vi "Teleop.vi"(10 "Match Info":T1={"Autonomous Elapsed Seconds"=0.0, "TeleOp Elapsed Seconds"=0.0, "Disabled Elapsed Seconds"=0.0, "Visited Autonomous"=FALSE, "Visited TeleOp"=FALSE, "Visited Disabled"=FALSE, "Autonomous Settings"={"Autonomous Style"=enum."Independent", "VI Refnum"=refnum}}, 11 "Call Context":T2) -> ()   [LabVIEW 2016]
doc: "This VI is called for each TeleOp packet received from the DS where the robot is not disabled. It is often used to read from the joysticks and update I/O or to update setpoints for timed control loops. It should complete and return within 20 milliseconds or it may miss DS packets."
uses:
  <vilib>/Rock Robotics/WPI/Ultrasonic/WPI_SonarSRF04DigitalRefNum Registry Get.vi
  <vilib>/Rock Robotics/WPI/Ultrasonic/WPI_SonarSRF04DigitalGetRange.vi
  <vilib>/gmath/NI_Gmath.lvlib
  <vilib>/Rock Robotics/WPI/Relay/WPI_RelayValue.ctl
  <vilib>/Rock Robotics/WPI/DriverStation/WPI_DriverStationMatch Info.ctl
  <vilib>/Rock Robotics/WPI/DriverStation/WPI_DriverStationDerivedRobotMode.ctl
panel:
  in  "Control Effort":dbl[](array[numeric])=[0.0, 0.0, 0.0, 0.0]
  in  "RPM Array":dbl[](array[numeric])=[0.0, 0.0, 0.0, 0.0]
  out "Encoder Index Count":dbl
  in  "OR Speed":dbl
  in  "Override?":bool
  out "Shooter RPM":dbl
  in  "kP":dbl=1.0 format="%#_13g"
  out "Shooter RPM 2":dbl(graph)
  in  "SET RPM":dbl format="%#_13g"
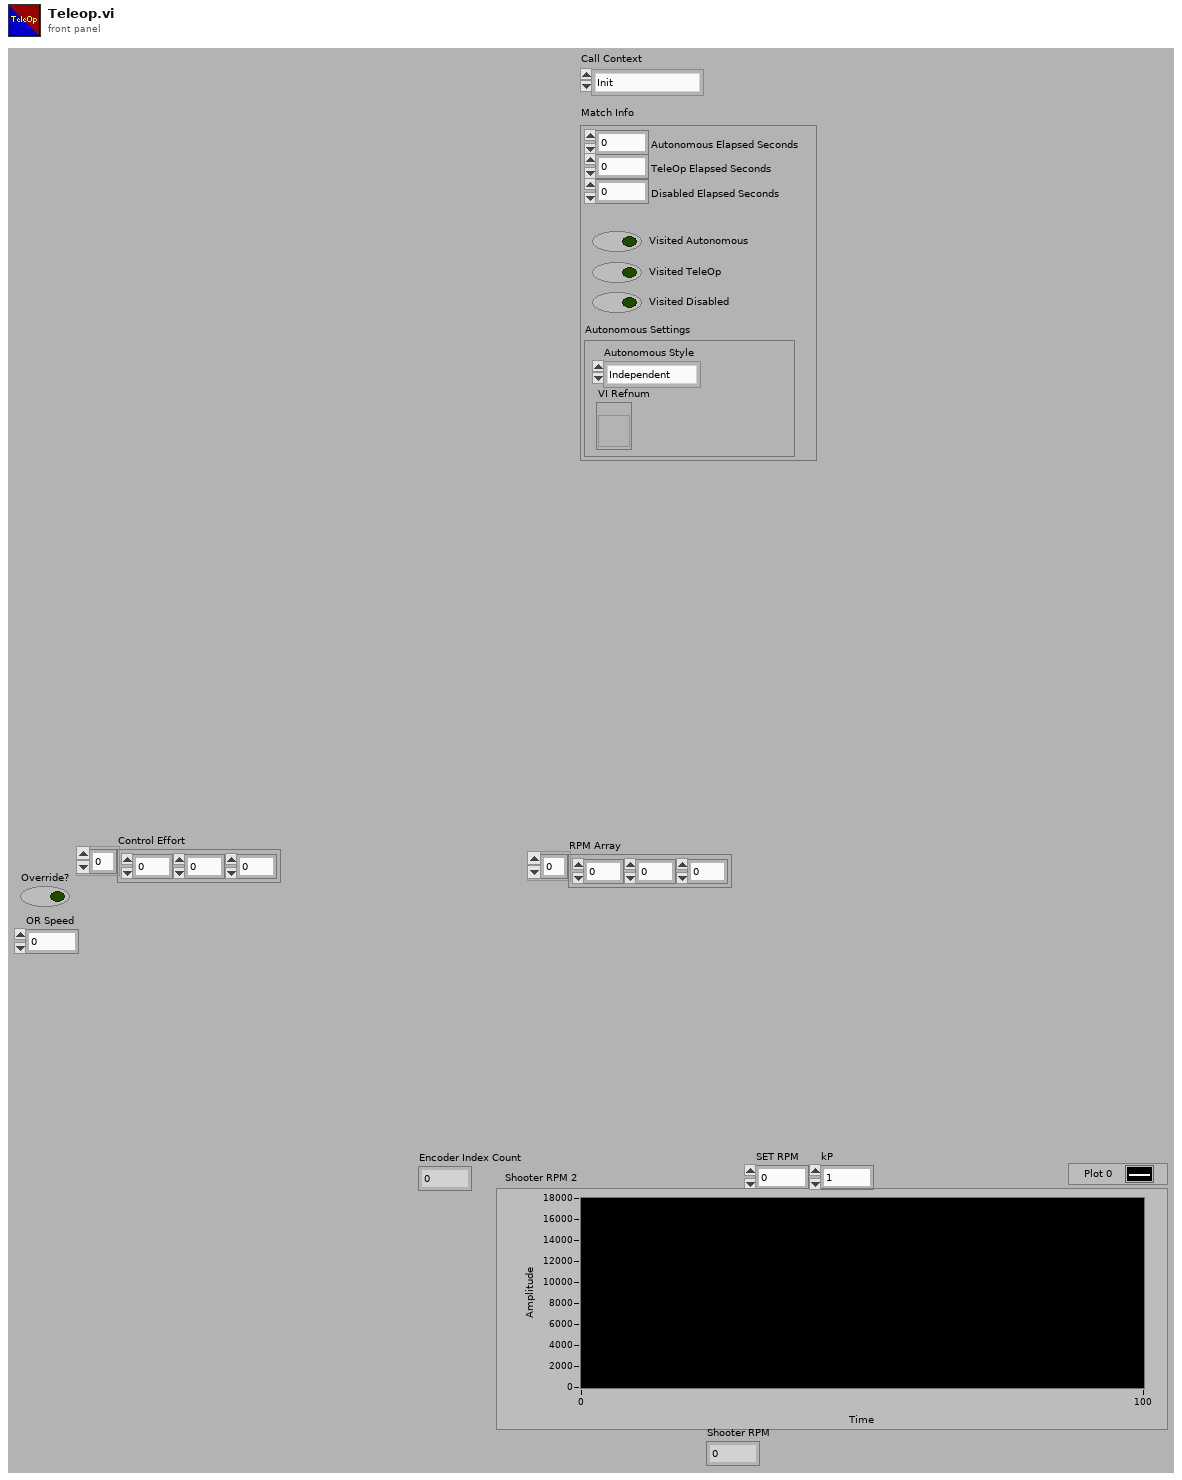
[diagram p1: front panel]
types:
  T1 = typedef "WPI_DriverStationMatch Info.ctl" = cluster{"Autonomous Elapsed Seconds":dbl, "TeleOp Elapsed Seconds":dbl, "Disabled Elapsed Seconds":dbl, "Visited Autonomous":bool, "Visited TeleOp":bool, "Visited Disabled":bool, "Autonomous Settings":cluster{"Autonomous Style":enum16{"Iterative", "Independent"}, "VI Refnum":refnum<vi>}}
  T2 = typedef "WPI_DriverStationDerivedRobotMode.ctl" = enum16{"Init", "Execute", "Stop"}
  T3 = typedef "WPI_JoystickDevRef.ctl" = cluster{"Device":T4}
  T4 = typedef "WPI_JoystickDeviceEnum.ctl" = enum16{"USB 0", "USB 1", "USB 2", "USB 3", "USB 4", "USB 5"}
  T5 = typedef "WPI_MotorControlDeviceRef.ctl" = cluster{"DeviceStatus":errorcluster, "Type":T6, "PWM":cluster{"PWM Channel":T7, "DeadBand":T8}, "CAN":cluster{"Device Number":u8, "SetOutput VI Ref":variant, "GetOutput VI Ref":variant, "Enable VI Ref":variant, "Disable VI Ref":variant, "Data":variant}, "Invert":bool}
  T6 = typedef "WPI_MotorControlType.ctl" = enum16{"PWM", "CAN"}
  T7 = typedef "FPGA_DIOPWMChannel.ctl" = enum8{"PWM 0", "PWM 1", "PWM 2", "PWM 3", "PWM 4", "PWM 5", "PWM 6", "PWM 7", "PWM 8", "PWM 9", "PWM MXP 0", "PWM MXP 1", "PWM MXP 2", "PWM MXP 3", "PWM MXP 4", "PWM MXP 5", "PWM MXP 6", "PWM MXP 7", "PWM MXP 8", "PWM MXP 9", "Invalid"}
  T8 = typedef "WPI_PWMDeadband.ctl" = cluster{"Name":string, "maxPositivePwm":i32, "minPositivePwm":i32, "centerPwm":i32, "maxNegativePwm":i32, "minNegativePwm":i32, "angularRange":u16}
  T9 = typedef "WPI_CANTalonSRX_GlobalStatus.ctl" = cluster{"Applied Throttle":dbl, "Module Enabled":bool, "CAN Error":errorcluster, "Closed Loop Error":dbl, "Forward Limit Switch Closed":bool, "Reverse Limit Switch Closed":bool, "Sensor Position":dbl, "Sensor Velocity":dbl, "Current":dbl, "Sticky Fault - Over Temp":bool, "Sticky Fault - Under Voltage":bool, "Sticky Fault - Forward Limit":bool, "Sticky Fault - Reverse Limit":bool, "Sticky Fault - Forward Soft Limit":bool, "Sticky Fault - Reverse Soft Limit":bool, "Brake is Enabled":bool, "Encoder Position":dbl, "Encoder Velocity":dbl, "Encoder Index Count":dbl, "Encoder A Pin State":bool, "Encoder B Pin State":bool, "Encoder Index Pin State":bool, "Analog In":dbl, "Analog In Velocity":dbl, "Temperature (C)":dbl, "Battery Voltage":dbl, "Control 5 Is Supported":bool, "Current Profile Slot Select":dbl, "Pos Div 8":bool, "Vel Div 4":bool, "Pulse Width Position":i32, "Pulse Width Velocity":i32, "Pulse Width Rise To Rise (us)":i32, "Pulse Width Rise To Fall (us)":i32, "Mot Prof Active Is Under Run":bool, "Mot Prof Active Has Under Run":bool, "Mot Prof Active Is Last":bool, "Mot Prof Active Velocity Only":bool, "Mot Prof Active Is Valid":bool, "Mot Prof Buffer Is Full":bool, "Mot Prof Active Profile Slot Select":i32, "Mot Prof NextID":i32, "Mot Prof Count":i32, "Mot Prof Active Velocity":dbl, "Mot Prof Active Position":dbl, "Mot Prof Output Enable":i32}
  T10 = typedef "WPI_UltrasonicDeviceRef.ctl" = cluster{"DevStatus":errorcluster, "Ping Channel":T11, "Echo Channel":T11, "CntIndex":T12}
  T11 = typedef "FPGA_DIOChannel.ctl" = enum8{"DIO 0", "DIO 1", "DIO 2", "DIO 3", "DIO 4", "DIO 5", "DIO 6", "DIO 7", "DIO 8", "DIO 9", "DIO MXP 0", "DIO MXP 1", "DIO MXP 2", "DIO MXP 3", "DIO MXP 4", "DIO MXP 5", "DIO MXP 6", "DIO MXP 7", "DIO MXP 8", "DIO MXP 9", "DIO MXP 10", "DIO MXP 11", "DIO MXP 12", "DIO MXP 13", "DIO MXP 14", "DIO MXP 15", "SPI Port CS1", "SPI Port CS2", "SPI Port CS3", "SPI Port MISO", "SPI Port MOSI", "Invalid"}
  T12 = typedef "FPGA_CounterCtrSystemIndex.ctl" = enum8{"Ctr 0", "Ctr 1", "Ctr 2", "Ctr 3", "Ctr 4", "Ctr 5", "Ctr 6", "Ctr 7", "Invalid"}
  T13 = typedef "WPI_GyroDevRef.ctl" = cluster{"DevStatus":errorcluster, "Analog Channel":T14, "Offset":dbl, "Gain (VoltsPerDegree/Second)":dbl, "Gyro Type":enum16{"Analog", "XRS450"}, "Handle":i32, "SPI Bus":T15, "Device Found":bool, "Sample Rate":dbl, "Calibrate On Open":bool}
  T14 = typedef "FPGA_AIChannel.ctl" = enum8{"AI 0", "AI 1", "AI 2", "AI 3", "AI MXP 0", "AI MXP 1", "AI MXP 2", "AI MXP 3", "Invalid"}
  T15 = typedef "spi_bus.ctl" = enum16{"SPI On-Board, CS0", "SPI On-Board, CS1", "SPI On-Board, CS2", "SPI On-Board, CS3", "SPI MXP", "Invalid"}
  T16 = typedef "WPI_RelayValue.ctl" = enum16{"Off", "On", "Forward", "Reverse"}
  T17 = typedef "WPI_RelayDevRef.ctl" = cluster{"DevStatus":errorcluster, "Relay Channel":T18, "Relay Direction":T19}
  T18 = typedef "FPGA_DIORelayChannel.ctl" = enum8{"Relay 0", "Relay 1", "Relay 2", "Relay 3", "Invalid"}
  T19 = typedef "WPI_RelayDirection.ctl" = enum16{"Both directions", "Forward only", "Reverse only"}
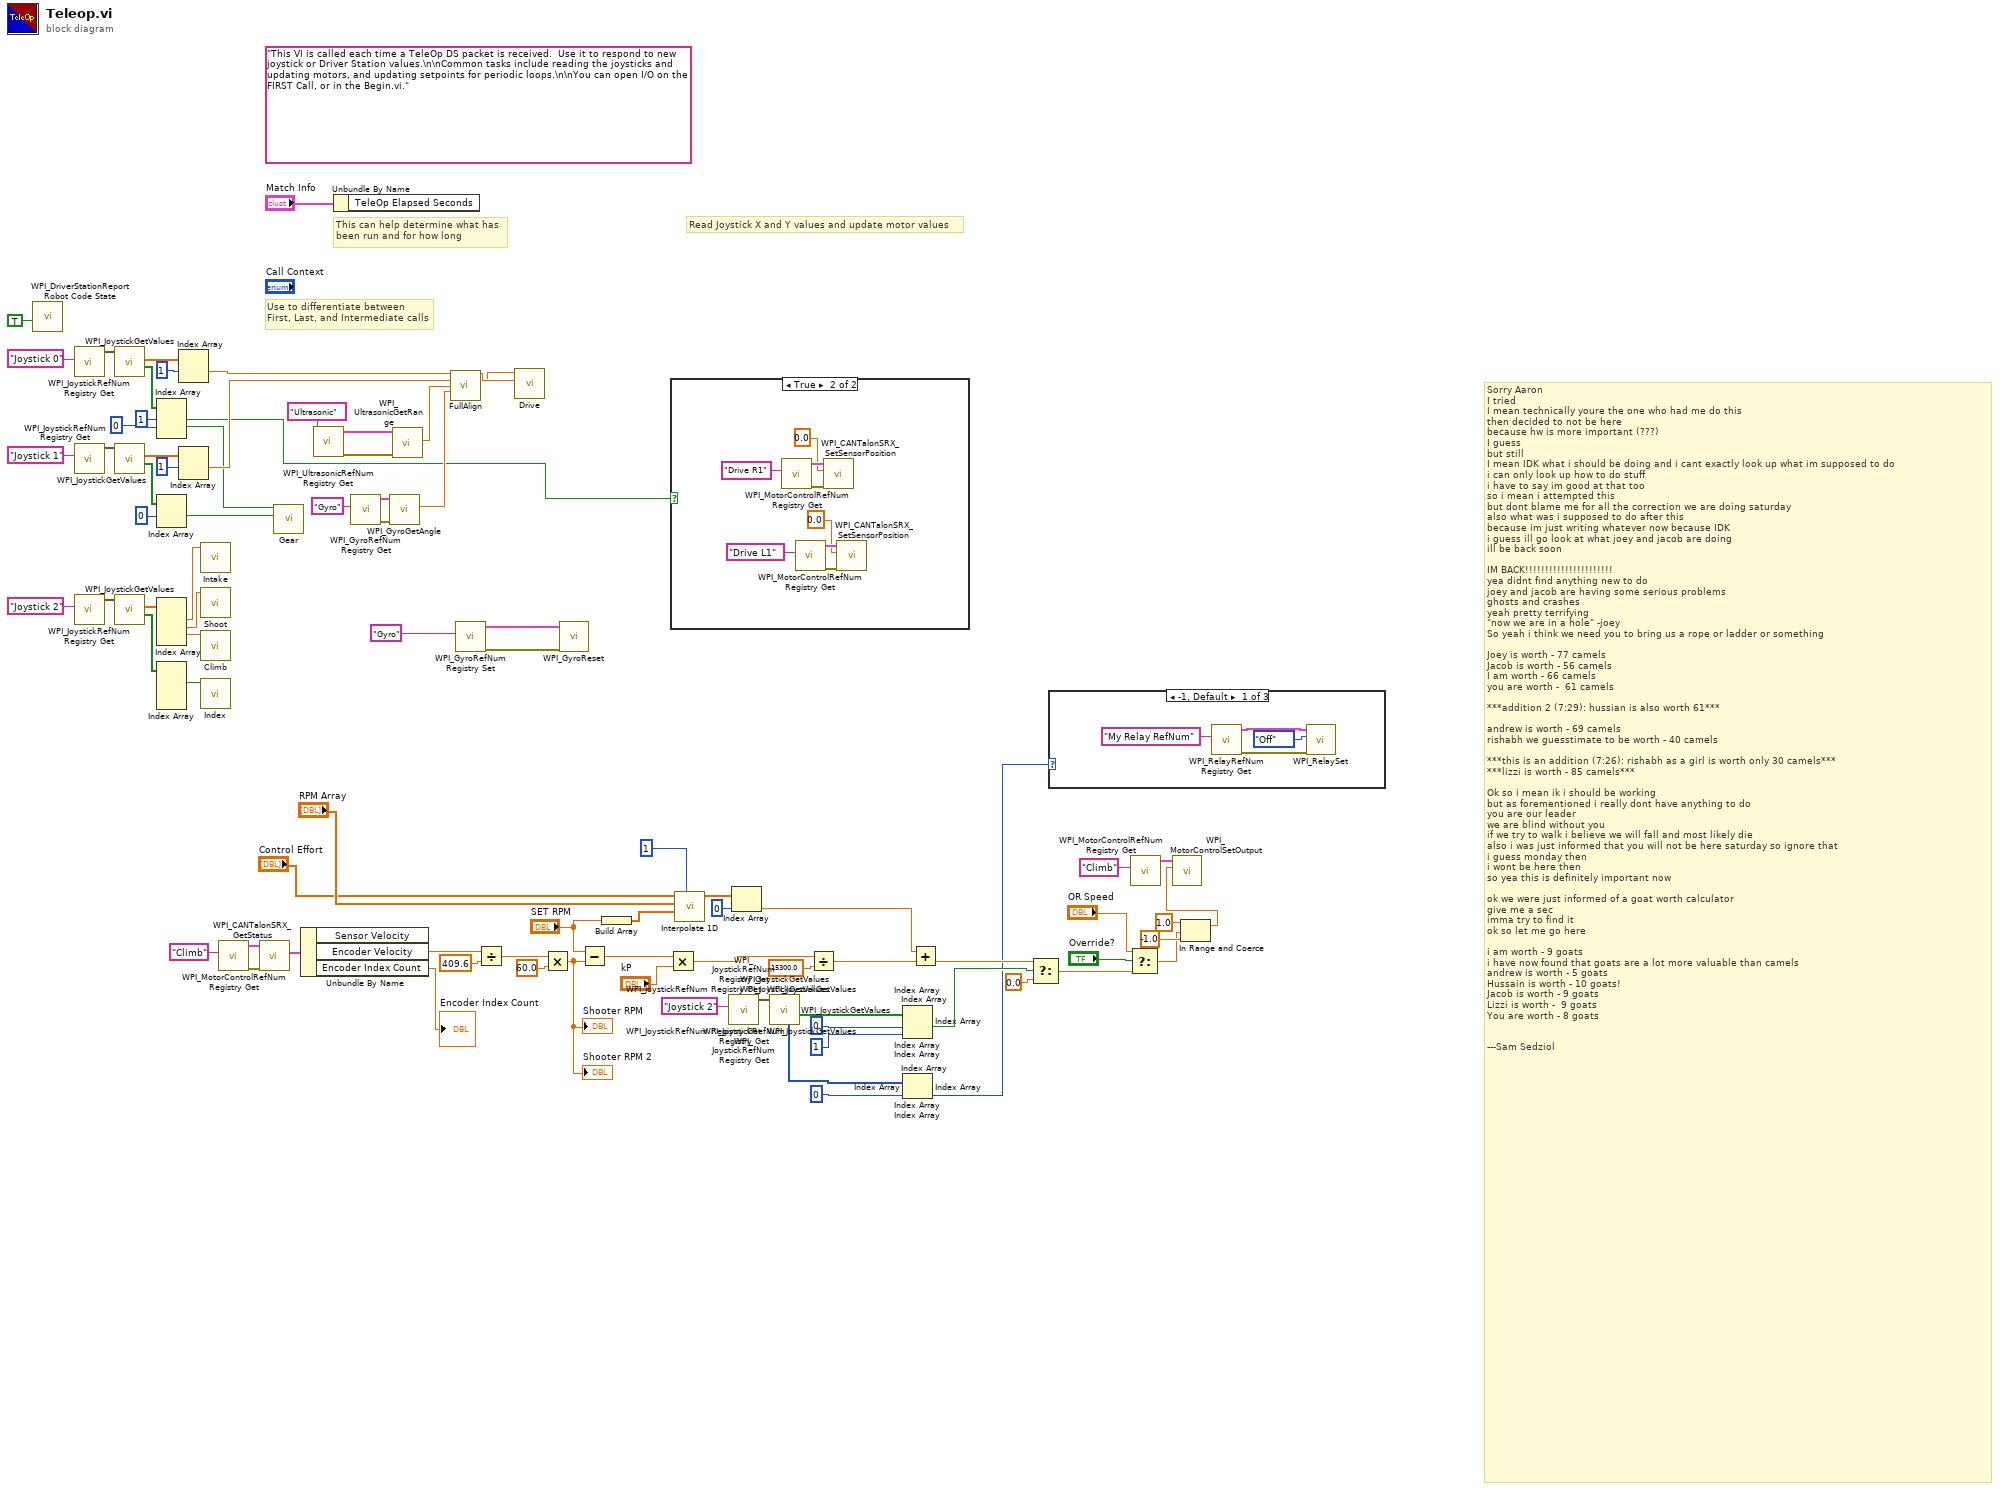
[diagram p0: block diagram]
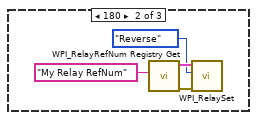
[diagram p3: hidden frame]
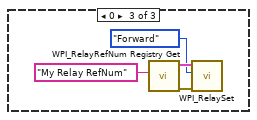
[diagram p4: hidden frame]
diagram:
  (unwired) "This VI is called each time a TeleOp DS packet is received.  Use it to respond to new joystick or Driver Station values.\n\nCommon tasks include reading the joysticks and updating motors, and updating setpoints for periodic loops.\n\nYou can open I/O on the FIRST Call, or in the Begin.vi."
  # "Sorry Aaron\nI tried\nI mean technically youre the one who had me do this\nthen decided to not be here\nbecause hw is more important (???)\nI guess\nbut still\nI mean IDK what i should be doing and i cant exactly look up what im supposed to do\ni can only look up how to do stuff\ni have to say im good at that too\nso i mean i attempted this\nbut dont blame me for all the correction we are doing saturday\nalso what was i supposed to do after this\nbecause im just writing whatever now because IDK\ni guess ill go look at what joey and jacob are doing\nill be back soon\n\nIM BACK!!!!!!!!!!!!!!!!!!!!!!\nyea didnt find anything new to do\njoey and jacob are having some serious problems\nghosts and crashes\nyeah pretty terrifying\n\"now we are in a hole\" -joey\nSo yeah i think we need you to bring us a rope or ladder or something\n\nJoey is worth - 77 camels\nJacob is worth - 56 camels\nI am worth - 66 camels\nyou are worth -  61 camels \n\n***addition 2 (7:29): hussian is also worth 61***\n\nandrew is worth - 69 camels\nrishabh we guesstimate to be worth - 40 camels\n\n***this is an addition (7:26): rishabh as a girl is worth only 30 camels***\n***lizzi is worth - 85 camels***\n\nOk so i mean ik i should be working\nbut as forementioned i really dont have anything to do\nyou are our leader\nwe are blind without you\nif we try to walk i believe we will fall and most likely die\nalso i was just informed that you will not be here saturday so ignore that\ni guess monday then\ni wont be here then\nso yea this is definitely important now\n\nok we were just informed of a goat worth calculator\ngive me a sec \nimma try to find it\nok so let me go here\n\ni am worth - 9 goats\ni have now found that goats are a lot more valuable than camels\nandrew is worth - 5 goats\nHussain is worth - 10 goats! \nJacob is worth - 9 goats\nLizzi is worth -  9 goats\nYou are worth - 8 goats\n\n\n---Sam Sedziol"
  # "Use to differentiate between\nFirst, Last, and Intermediate calls"
  # "This can help determine what has\nbeen run and for how long"
  # "Read Joystick X and Y values and update motor values"
  n1 = call <vilib>:"WPI_DriverStationReport Robot Code State.vi"("TeleOp"=TRUE ("Autonomous")) -> ()  [unwired: 10 in, 1 out]
  n2 = call <vilib>:"WPI_JoystickRefNum Registry Get.vi"("refnum name"="Joystick 0") -> ("JoystickDevRef"=w111:T3)  [unwired: 1 in, 9 out]
  n3 = call <vilib>:"WPI_JoystickRefNum Registry Get.vi"("refnum name"="Joystick 1") -> ("JoystickDevRef"=w107:T3)  [unwired: 1 in, 9 out]
  n4 = call <vilib>:"WPI_JoystickRefNum Registry Get.vi"("refnum name"="Joystick 2") -> ("JoystickDevRef"=w104:T3)  [unwired: 1 in, 9 out]
  n5 = call <vilib>:"WPI_JoystickGetValues.vi"("JoystickDevRef"=w111) -> ("Buttons"=w100:bool[], "Axes"=w109:dbl[])  [unwired: 6 in, 3 out]
  n6 = call <vilib>:"WPI_JoystickGetValues.vi"("JoystickDevRef"=w107) -> ("Buttons"=w101:bool[], "Axes"=w108:dbl[])  [unwired: 6 in, 3 out]
  n7 = call <vilib>:"WPI_JoystickGetValues.vi"("JoystickDevRef"=w104) -> ("Buttons"=w102:bool[], "Axes"=w103:dbl[])  [unwired: 6 in, 3 out]
  n8 = Index Array(array=w100, index #1=1 ("index"), index #2=0 ("index")) -> (element #1=w9:bool, element #2=w7:bool)  [unwired: 1 in, 1 out]
  n9 = Index Array(array=w101, index #1=0 ("index")) -> (element #1=w6:bool)  [unwired: 1 in, 1 out]
  n10 = Index Array(array=w103) -> (element #1=w95:dbl, element #2=w96:dbl, element #3=w94:dbl)  [unwired: 4 in, 1 out]
  n11 = Index Array(array=w102) -> (element #1=w93:bool)  [unwired: 4 in, 3 out]
  n12 = Index Array(array=w109, index #1=1 ("index")) -> (element #1=w90:dbl)  [unwired: 1 in, 1 out]
  n13 = Index Array(array=w108, index #1=1 ("index")) -> (element #1=w89:dbl)  [unwired: 1 in, 1 out]
  n14 = call "Intake.vi"("Effort"=w95) -> ()  [unwired: 11 in]
  n15 = call "Shoot.vi"("Effort"=w96) -> ()  [unwired: 11 in]
  n16 = call "Climb.vi"("Effort"=w94) -> ()  [unwired: 11 in]
  n17 = call "Index.vi"("Index?"=w93) -> ()  [unwired: 11 in]
  n18 = call <vilib>:"WPI_MotorControlRefNum Registry Get.vi"("refnum name"="Climb") -> ("error out"=w30:errorcluster, "MotorControlDevRef"=w29:T5)  [unwired: 9 in]
  n19 = call <vilib>:"WPI_CANTalonSRX_GetStatus.vi"("error in (no error)"=w30, "CAN Talon SRX Ref"=w29) -> ("Talon SRX Status"=w39:T9)  [unwired: 7 in, 2 out]
  n20 = call "Gear.vi"("Gear1?"=w6, "Gear0?"=w7) -> ()  [unwired: 10 in]
  n21 = Unbundle By Name(w39) -> ("Encoder Velocity"=w33:dbl, "Encoder Index Count"=→"Encoder Index Count":dbl)  [unwired: 1 out]
  n22 = call-poly <vilib>:"WPI_UltrasonicRefNum Registry Get.vi"("refnum name"="Ultrasonic") -> ("error out"=w83:errorcluster, "SonarSRF04DevRef"=w84:T10)  [unwired: 9 in]
  n23 = Unbundle By Name("Match Info") -> ()  [unwired: 1 out]
  n24 = call <vilib>:"WPI_GyroRefNum Registry Get.vi"("refnum name"="Gyro") -> ("error out"=w88:errorcluster, "GyroDevRef"=w87:T13)  [unwired: 9 in]
  n25 = call <vilib>:"WPI_GyroGetAngle.vi"("error in"=w88, "GyroDevRef"=w87) -> ("Angle"=w85:dbl)  [unwired: 5 in, 4 out]
  n26 = call-poly <vilib>:"WPI_UltrasonicGetRange.vi"("error in (no error)"=w83, "SonarSRF04DevRef"=w84) -> ("Distance"=w81:dbl)  [unwired: 7 in, 2 out]
  n27 = call "FullAlign.vi"("Joystick 0"=w90, "Joystick 1"=w89, "Distance"=w81, "Angle"=w85) -> ("Right Motor"=w92:dbl, "Left Motor"=w91:dbl)  [unwired: 7 in, 3 out]
  n28 = call <vilib>:"WPI_GyroRefNum Registry Set.vi"("refnum name"="Gyro") -> ("error out"=w2:errorcluster, "GyroDevRef"=w3:T13)  [unwired: 9 in]
  n29 = Divide(x=w33, y=409.6) -> (x/y=w32:dbl)
  n30 = call "Drive.vi"("Drive R"=w92, "Drive L"=w91) -> ()  [unwired: 10 in]
  n31 = Multiply(x=w32, y=60.0) -> (x*y=w35:dbl)
  "Shooter RPM 2" <- w35
  "Shooter RPM" <- w35
  n32 = call <vilib>:"WPI_GyroReset.vi"("error in"=w2, "GyroDevRef"=w3) -> ()  [unwired: 8 in, 2 out]
  n33 = Subtract(x="SET RPM", y=w35) -> (x-y=w20:dbl)
  n34 = Build Array("SET RPM") -> (w44:dbl[])
  n35 = Multiply(x=w20, y="kP") -> (x*y=w38:dbl)
  n36 = case shown="True" w9 {
    frame False {
    }
    frame True {
      n37 = call <vilib>:"WPI_MotorControlRefNum Registry Get.vi"("refnum name"="Drive R1") -> ("error out"=w115:errorcluster, "MotorControlDevRef"=w114:T5)  [unwired: 9 in]
      n38 = call <vilib>:"WPI_MotorControlRefNum Registry Get.vi"("refnum name"="Drive L1") -> ("error out"=w117:errorcluster, "MotorControlDevRef"=w118:T5)  [unwired: 9 in]
      n39 = call <vilib>:"WPI_CANTalonSRX_SetSensorPosition.vi"("error in (no error)"=w115, "New Sensor Position"=0.0, "CAN Talon SRX Ref"=w114) -> ()  [unwired: 7 in, 2 out]
      n40 = call <vilib>:"WPI_CANTalonSRX_SetSensorPosition.vi"("error in (no error)"=w117, "New Sensor Position"=0.0, "CAN Talon SRX Ref"=w118) -> ()  [unwired: 7 in, 2 out]
    }
  }
  n41 = call <vilib>:"Interpolate 1D.vi"("method"=1, "xi"=w44, "X"="RPM Array", "Y"="Control Effort") -> ("yi"=w45:dbl[])  [unwired: 5 in, 2 out]
  n42 = call <vilib>:"WPI_JoystickRefNum Registry Get.vi"("refnum name"="Joystick 2") -> ("JoystickDevRef"=w79:T3)  [unwired: 1 in, 9 out]
  n43 = call <vilib>:"WPI_JoystickRefNum Registry Get.vi"("refnum name"="Joystick 2") -> ("JoystickDevRef"=w72:T3)  [unwired: 1 in, 9 out]
  n44 = call <vilib>:"WPI_JoystickRefNum Registry Get.vi"("refnum name"="Joystick 2") -> ("JoystickDevRef"=w61:T3)  [unwired: 1 in, 9 out]
  n45 = call <vilib>:"WPI_JoystickRefNum Registry Get.vi"("refnum name"="Joystick 2") -> ("JoystickDevRef"=w58:T3)  [unwired: 1 in, 9 out]
  n46 = call <vilib>:"WPI_JoystickRefNum Registry Get.vi"("refnum name"="Joystick 2") -> ("JoystickDevRef"=w15:T3)  [unwired: 1 in, 9 out]
  n47 = Index Array(array=w45, index=0) -> (element=w48:dbl)
  n48 = call <vilib>:"WPI_JoystickGetValues.vi"("JoystickDevRef"=w79) -> ("Buttons"=w77:bool[], "POVs"=w74:i16[])  [unwired: 6 in, 3 out]
  n49 = call <vilib>:"WPI_JoystickGetValues.vi"("JoystickDevRef"=w72) -> ("Buttons"=w70:bool[], "POVs"=w67:i16[])  [unwired: 6 in, 3 out]
  n50 = call <vilib>:"WPI_JoystickGetValues.vi"("JoystickDevRef"=w61) -> ("Buttons"=w63:bool[], "POVs"=w66:i16[])  [unwired: 6 in, 3 out]
  n51 = call <vilib>:"WPI_JoystickGetValues.vi"("JoystickDevRef"=w58) -> ("Buttons"=w56:bool[], "POVs"=w53:i16[])  [unwired: 6 in, 3 out]
  n52 = call <vilib>:"WPI_JoystickGetValues.vi"("JoystickDevRef"=w15) -> ("Buttons"=w17:bool[], "POVs"=w23:i16[])  [unwired: 6 in, 3 out]
  n53 = Divide(x=w38, y=15300.0) -> (x/y=w37:dbl)
  n54 = Index Array(array=w77, index #1=0 ("index"), index #2=1 ("index")) -> (element #1=w11:bool)  [unwired: 1 out]
  n55 = Index Array(array=w70, index #1=0 ("index"), index #2=1 ("index")) -> ()  [unwired: 2 out]
  n56 = Index Array(array=w63, index #1=0 ("index"), index #2=1 ("index")) -> ()  [unwired: 2 out]
  n57 = Index Array(array=w56, index #1=0 ("index"), index #2=1 ("index")) -> ()  [unwired: 2 out]
  n58 = Index Array(array=w17, index #1=0 ("index"), index #2=1 ("index")) -> ()  [unwired: 2 out]
  n59 = Index Array(array=w74, index=0) -> (element=w10:i16)
  n60 = Index Array(array=w67, index=0) -> ()  [unwired: 1 out]
  n61 = Index Array(array=w66, index=0) -> ()  [unwired: 1 out]
  n62 = Index Array(array=w53, index=0) -> ()  [unwired: 1 out]
  n63 = Index Array(array=w23, index=0) -> ()  [unwired: 1 out]
  n64 = Add(x=w48, y=w37) -> (x+y=w47:dbl)
  n65 = Select(t=w47, s=w11, f=0.0) -> (s? t:f=w27:dbl)
  n66 = case shown="-1, Default" w10 {
    frame -1, Default {
      n67 = call <vilib>:"WPI_RelayRefNum Registry Get.vi"("refnum name"="My Relay RefNum") -> ("error out"=w124:errorcluster, "RelayDevRef"=w123:T17)  [unwired: 9 in]
      n68 = call <vilib>:"WPI_RelaySet.vi"("error in (no error)"=w124, "RelayValue"=WPI_RelayValue."Off", "RelayDevRef"=w123) -> ()  [unwired: 7 in, 2 out]
    }
    frame 180 {
      n69 = call <vilib>:"WPI_RelayRefNum Registry Get.vi"("refnum name"="My Relay RefNum") -> ("error out"=w128:errorcluster, "RelayDevRef"=w127:T17)  [unwired: 9 in]
      n70 = call <vilib>:"WPI_RelaySet.vi"("error in (no error)"=w128, "RelayValue"=WPI_RelayValue."Reverse", "RelayDevRef"=w127) -> ()  [unwired: 7 in, 2 out]
    }
    frame 0 {
      n71 = call <vilib>:"WPI_RelayRefNum Registry Get.vi"("refnum name"="My Relay RefNum") -> ("error out"=w132:errorcluster, "RelayDevRef"=w131:T17)  [unwired: 9 in]
      n72 = call <vilib>:"WPI_RelaySet.vi"("error in (no error)"=w132, "RelayValue"=WPI_RelayValue."Forward", "RelayDevRef"=w131) -> ()  [unwired: 7 in, 2 out]
    }
  }
  n73 = Select(t="OR Speed", s="Override?", f=w27) -> (s? t:f=w49:dbl)
  n74 = call <vilib>:"WPI_MotorControlRefNum Registry Get.vi"("refnum name"="Climb") -> ("MotorControlDevRef"=w12:T5)  [unwired: 9 in, 1 out]
  n75 = In Range and Coerce(upper limit=1.0, x=w49, lower limit=-1.0) -> (coerced(x)=w52:dbl)  [unwired: 1 out]
  n76 = call <vilib>:"WPI_MotorControlSetOutput.vi"("Output"=w52, "MotorControlDevRef"=w12) -> ()  [unwired: 7 in, 3 out]
